vi "Get Userdefined Symbol.vi"(8 "错误输入":errorcluster, 10 "Index":i32, 11 "Listbox Ref":refnum<vi>) -> (0 "错误输出":errorcluster, 2 "Image":T1 caption="图像", 3 "Dup Listbox Ref":refnum<vi>)   [LabVIEW 2011, in "Listbox Tool.lvlib"]
uses:
  Listbox Tool.lvlib
  <vilib>/picture/picture.llb/imagedata.ctl
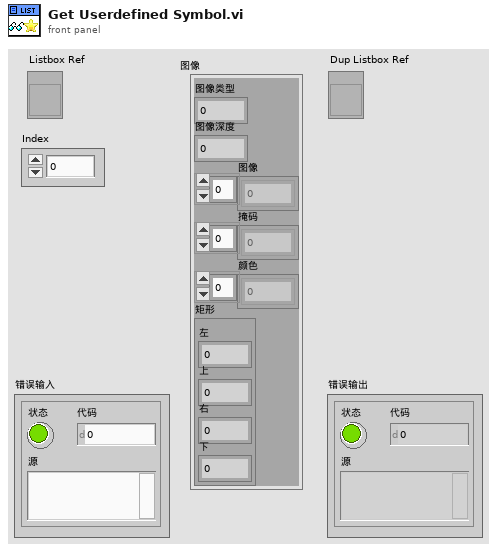
[diagram p1: front panel]
types:
  T1 = typedef "imagedata.ctl" = cluster{"image type":i32, "image depth":i32, "image":u8[], "mask":u8[], "colors":u32[], "Rectangle":cluster{"left":i16, "top":i16, "right":i16, "bottom":i16}}
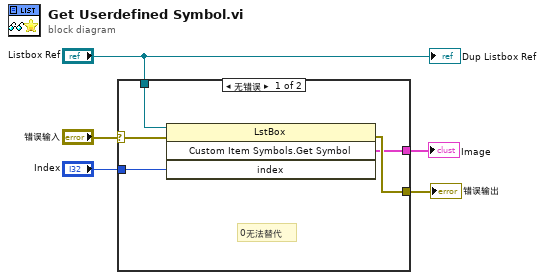
[diagram p0: block diagram]
diagram:
  n1 = case shown="无错误" "错误输入" {
    selector: "错误输入" -> [w9 w11]
    tunnel: [w8 w11] -> w4
    tunnel: "Listbox Ref" -> [w10 _]
    tunnel: "Index" -> [w7 _]
    tunnel: [w6 _] -> w1
    frame No Error {
      # "0无法替代"
      n2 = invoke class="LstBox" method="Custom Item Symbols.Get Symbol"(reference=w10, error in=w9, "index"=w7) -> (error out=w8:errorcluster, "Custom Item Symbols:Get Symbol"=w6:T1)  [unwired: 1 in, 2 out]
    }
    frame Error {
    }
  }
  "错误输出" <- w4
  "Image" <- w1
  "Dup Listbox Ref" <- "Listbox Ref"
